vi "VI-Create KObject Dialog.vi"() -> ()   [LabVIEW 2020]
uses:
  Buttons/KCheckmarkBoolean 2.ctl
panel:
  out "exit":bool
  in  "NewClass":T2={"Folder"=path "D:/Experiment VIs", "Name"="New Class", "New base class?"=FALSE, "Inherit from"=path "D:/Development/epl-vi-lib/Koop/KObject Class/KObject.lvclass"}
  in  "Create Class":bool
  # "KObject"
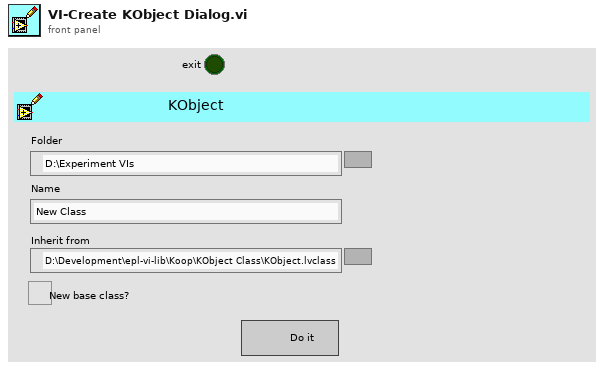
[diagram p1: front panel]
types:
  T1 = typedef "KCheckmarkBoolean 2.ctl" = bool
  T2 = cluster{"Folder":path, "Name":string, "New base class?":T1, "Inherit from":path}
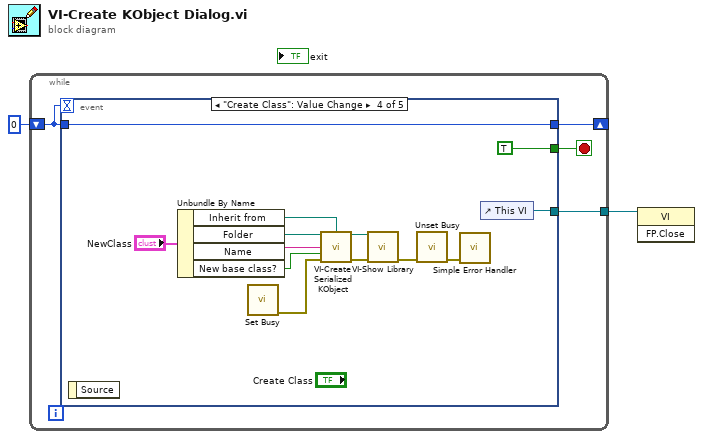
[diagram p0: block diagram]
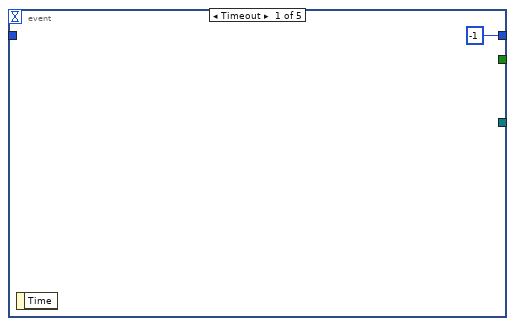
[diagram p2: hidden frame]
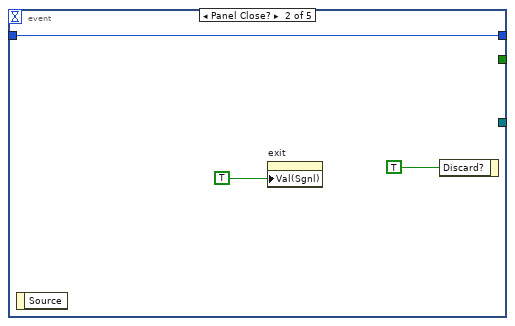
[diagram p3: hidden frame]
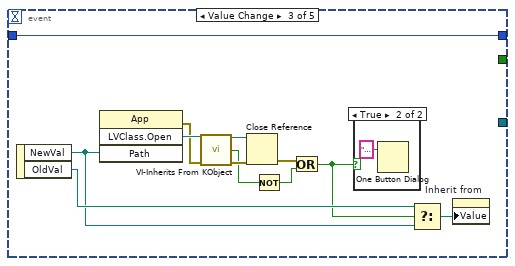
[diagram p4: hidden frame]
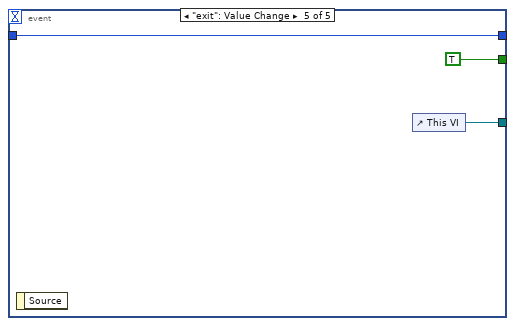
[diagram p6: hidden frame]
diagram:
  n1 = while {
    tunnel: [w6] -> w2
    shift-right: [w3] -> _
    shift-left: 0 -> [w4]
    stop <- w5 stop-if-true
    n2 = event shown="[3] \"Create Class\": Value Change" {
      selector: _ -> [_ _ _ _ _]
      dyn-events: _ -> [_ _ _ _ _]
      timeout: w4 -> [_ _ _ _ _]
      tunnel: [_ _ _ w34 w39] -> w6
      tunnel: [_ _ _ TRUE TRUE] -> w5
      tunnel: w4 -> [_ w8 w22 w31 w37]
      tunnel: [-1 w8 w22 w31 w37] -> w3
      event Timeout {
        n3 = event-data() -> ()  [unwired: 1 in, 1 out]
      }
      event Panel Close? {
        n4 = event-data() -> ()  [unwired: 1 in, 1 out]
        n5 = property on="exit" class="Bool (strict)"("Val(Sgnl)"=TRUE ("Value (Signaling)")) -> ()  [unwired: 2 in, 2 out]
        n6 = event-data("Discard?"=TRUE) -> ()  [unwired: 1 in, 1 out]
      }
      event "NewClass.Inherit from": Value Change {
        n7 = event-data() -> ("NewVal"=w12:path, "OldVal"=w13:path)  [unwired: 1 in]
        n8 = invoke class="App" method="LVClass.Open"("Path"=w12) -> (error out=w18:errorcluster, "LVClass.Open"=w21:refnum<vi>)  [unwired: 3 in, 2 out]
        n9 = call "VI-Inherits From KObject.vi"("LVClass Ref"=w21, "error in (no error)"=w18) -> ("LVClass Ref out"=w19:refnum<vi>, "inherits?"=w15:bool, "error out"=w20:errorcluster)  [unwired: 11 in]
        n10 = Close Reference(reference=w19, error in (no error)=w20) -> (error out=w16:errorcluster)
        n11 = Not(x=w15) -> (.not. x?=w14:bool)
        n12 = Or(x=w16, y=w14) -> (x .or. y?=w11:bool)
        n13 = case shown="True" w11 {
          frame False {
          }
          frame True {
            n14 = One Button Dialog(message="Not a serializable class!") -> ()  [unwired: 1 in, 1 out]
          }
        }
        n15 = Select(t=w13, s=w11, f=w12) -> (s? t:f=w17:path)
        n16 = property on="Inherit from" class="Path"("Value"=w17) -> ()  [unwired: 2 in, 2 out]
      }
      event "Create Class": Value Change {
        n17 = event-data() -> ()  [unwired: 1 in, 1 out]
        n18 = Unbundle By Name("NewClass") -> ("Inherit from"=w27:path, "Folder"=w30:path, "Name"=w33:string, "New base class?"=w32:T1)
        n19 = call <vilib>:"Set Busy.vi"() -> ("error out"=w29:errorcluster)  [unwired: 10 in, 1 out]
        n20 = call "VI-Create Serialized KObject.vi"("Folder"=w30, "Base class path"=w27, "Name"=w33, "Make base"=w32, "error in (no error)"=w29) -> ("Library"=w26:path, "error out"=w25:errorcluster)  [unwired: 9 in]
        n21 = call "VI-Show Library.vi"("Library Path"=w26, "error in (no error)"=w25) -> ("error out"=w24:errorcluster)  [unwired: 13 in]
        n22 = call <vilib>:"Unset Busy.vi"("error in (no error)"=w24) -> ("error out"=w28:errorcluster)  [unwired: 10 in]
        n23 = call <vilib>:"Simple Error Handler.vi"("error in (no error)"=w28) -> ()  [unwired: 4 in, 5 out]
        n24 = control-ref of="This VI"() -> (w34:refnum<vi>)
      }
      event "exit": Value Change {
        n25 = event-data() -> ()  [unwired: 1 in, 1 out]
        n26 = control-ref of="This VI"() -> (w39:refnum<vi>)
      }
    }
  }
  n27 = invoke class="VI" method="FP.Close"(reference=w2) -> ()  [unwired: 2 in, 3 out]
